vi "Test Basic DAQ.vi"() -> ()   [LabVIEW 2011, in "Diamond Universal Driver.lvlib"]
uses:
  Diamond Universal Driver.lvlib
  Controls/dscBool.ctl
  Controls/board type.ctl
  Controls/dsccb.ctl
  constants.vi
  Controls/gain.ctl
  Controls/dscADSettings.ctl
  Controls/state.ctl
  Controls/dscADScan.ctl
  Controls/dscPolarity.ctl
  Controls/dscDASettings.ctl
panel:
  out "error out 2":errorcluster
  out "error out":errorcluster
  out "LED V":dbl
  out "LED Curr":dbl
  out "P tot":dbl
  out "P up":dbl
  out "T Imp":dbl
  out "RH Imp":dbl
  out "T total":dbl
  out "RH Total":dbl
  out "T Upstream":dbl
  out "RH  Upstream":dbl
  out "purge flow":dbl
  out "sample flow":dbl
  out "sheath flow":dbl
  in  "LED On":bool
  in  "Inlet Temp":dbl
  in  "Purge Flow":dbl
  in  "Samp Flow":dbl
  in  "Sheath Flow":dbl
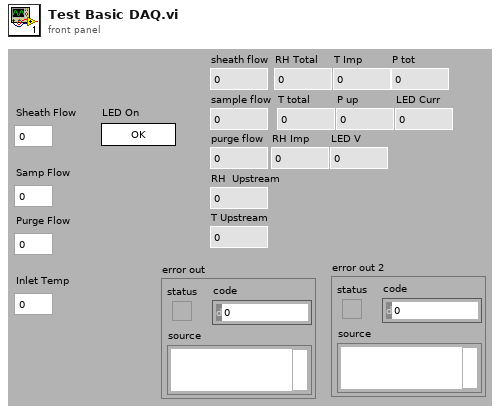
[diagram p1: front panel]
types:
  T1 = typedef "Diamond Universal Driver.lvlib/dscDASettings.ctl" = cluster{"polarity":T2, "load_cal":T3, "range":sgl, "Gain":enum16{"Gain of 1", "Gain of 2", "Gain of 4", "Gain of 8"}, "daSim":u8, "daPolEn":u8, "daUR":u8, "daURCh":u8}
  T2 = typedef "Diamond Universal Driver.lvlib/dscPolarity.ctl" = enum8{"BIPOLAR", "UNIPOLAR"}
  T3 = typedef "dscBool.ctl" = i32
  T4 = typedef "Diamond Universal Driver.lvlib/state.ctl" = enum16{"Sample", "Wait"}
  T5 = typedef "dscADSettings.ctl" = cluster{"current_ch":u8, "gain":T6, "range":enum8{"RANGE_5", "RANGE_10"}, "polarity":enum16{"BIPOLAR", "UNIPOLAR"}, "load cal":u8, "scan_int":enum8{"20", "15", "10", "5", "9", "4"}, "addiff":enum8{"Single Ended", "Differential"}}
  T6 = typedef "gain.ctl" = enum8{"GAIN_1", "GAIN_2", "GAIN_8"}
  T7 = typedef "board type.ctl" = u8
  T8 = typedef "dsccb.ctl" = cluster{"board type":T7, "board num":i16, "base addr":u16, "int level":u8, "RMM external trig":T3, "RMM external trig c3":T3, "EMM IOAdd":u16[], "EMM IOInterrupt":u16[], "clkfreq0":enum8{"10 MHz", "1 MHz"}, "clkfreq1":enum8{"10 MHz", "1 MHz"}, "clksel1":enum8{"Internal (clkfrq1)", "External"}, "address space":dbl, "DAC cfg":u8, "clck_freq":i32, "dma_level":u8, "int_lvl 1":u8, "int_lvl 2":u8, "int_lvl 3":u8, "fpga":u16, "smm_ad_res":u8, "RMM mode 16bit":T3, "RMM DAC 0_3 ext en":T3, "RMM DAC 4_7 ext en":T3}
  T9 = typedef "dscADScan.ctl" = cluster{"low channel":u8, "high channel":u8, "sample_val":u16[], "gain":T6}
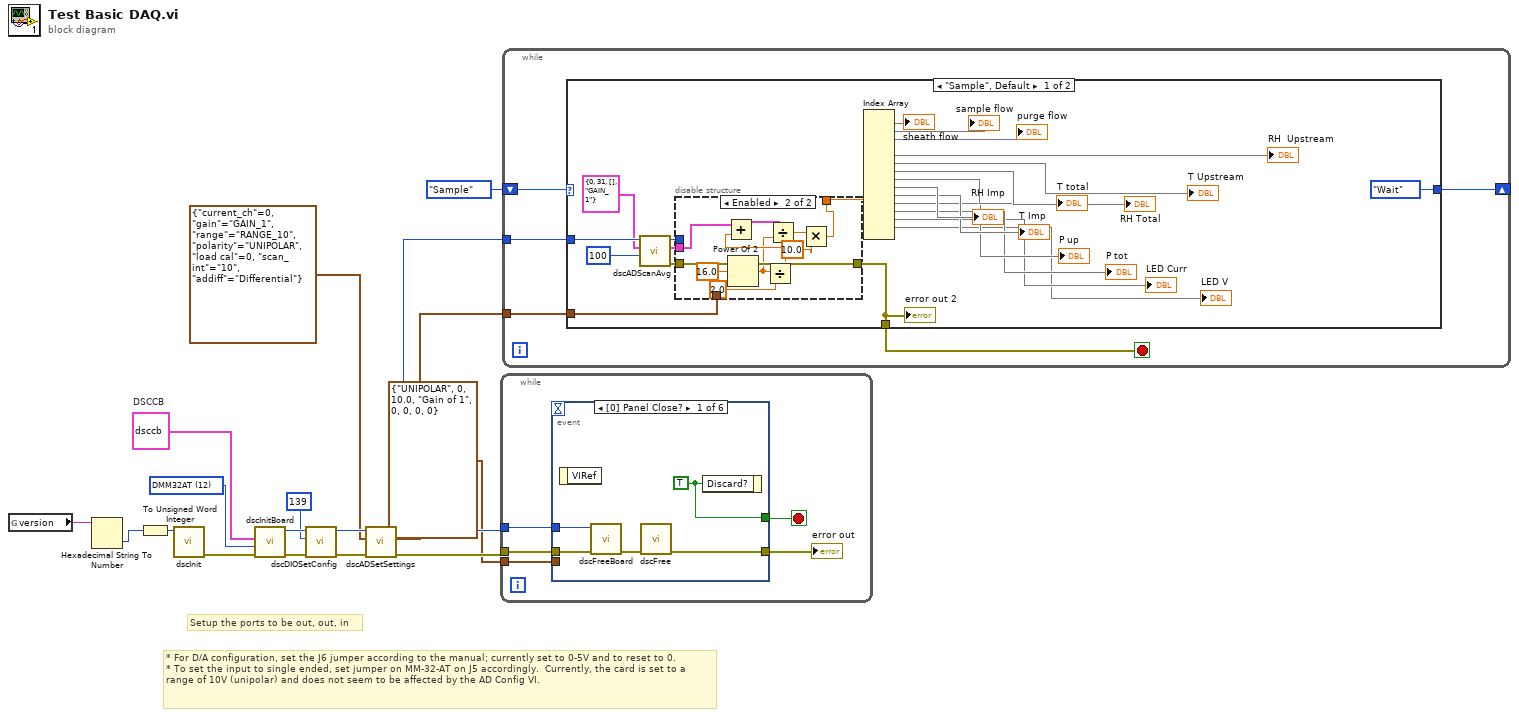
[diagram p0: block diagram]
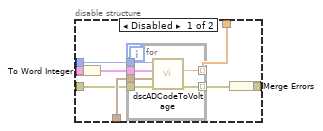
[diagram p2: hidden frame]
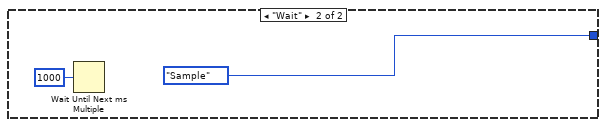
[diagram p3: hidden frame]
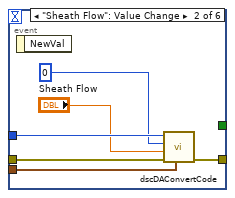
[diagram p4: hidden frame]
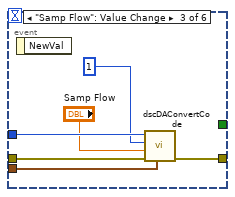
[diagram p5: hidden frame]
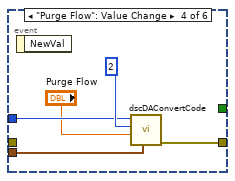
[diagram p6: hidden frame]
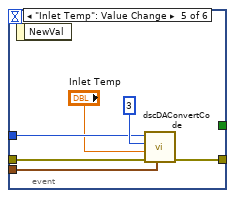
[diagram p7: hidden frame]
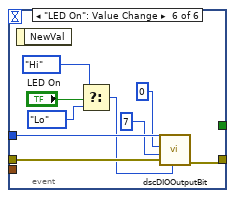
[diagram p8: hidden frame]
diagram:
  w13 = T7 12 items=["DMM16"=0, "RMM"=1, "TMM"=2, "OPMM"=3, "DMM"=4, "SMM"=5, "GMM"=6, "QMM"=7, "ZMM"=8, "PMM"=9, "OMM"=10, "RMM416"=11, "DMM32AT"=12, "EMMDIO"=13, "RMM1612"=14, "DMMAT"=15, "DMM16AT"=16, "IR104"=17, "EMM8"=18, "PROM"=19, "HERCEBX"=20, "CPT"=21, "DMM48AT"=22, "OMMIO"=23, "DIO82C55"=24, "ATHENA"=25, "METIS"=26, "DMM32XAT"=27, "ELEKTRA"=28, "GPIO11_9513"=29, "GPIO11_DIO"=30, "GPIO21"=31, "PSD"=32, "ATHENAII"=33, "DMM32DXAT"=34, "HELIOS"=35, "NEPTUNE"=36, "TEST"=126, "RAW"=127, "DRVR"=255] ("board type")
  w12 = T8 {"board type"=12, "board num"=1, "base addr"=768, "int level"=3, "RMM external trig"=0, "RMM external trig c3"=0, "EMM IOAdd"=[0, 0, 0, 0, 0, 0, 0, 0], "EMM IOInterrupt"=[0, 0, 0, 0, 0, 0, 0, 0], "clkfreq0"=enum."10 MHz", "clkfreq1"=enum."10 MHz", "clksel1"=enum."Internal (clkfrq1)", "address space"=0.0, "DAC cfg"=0, "clck_freq"=0, "dma_level"=0, "int_lvl 1"=0, "int_lvl 2"=0, "int_lvl 3"=0, "fpga"=0, "smm_ad_res"=0, "RMM mode 16bit"=0, "RMM DAC 0_3 ext en"=0, "RMM DAC 4_7 ext en"=0}  # DSCCB
  # "* For D/A configuration, set the J6 jumper according to the manual; currently set to 0-5V and to reset to 0.\n* To set the input to single ended, set jumper on MM-32-AT on J5 accordingly.  Currently, the card is set to a range of 10V (unipolar) and does not seem to be affected by the AD Config VI."
  # "Setup the ports to be out, out, in"
  n1 = global read "constants.vi" "version"() -> (w17:string)
  n2 = Hexadecimal String To Number(string=w17) -> (number=w15:u32)  [unwired: 2 in, 1 out]
  n3 = To Unsigned Word Integer(number=w15) -> (unsigned 16bit integer=w16:u16)
  n4 = call "dscInit.vi"("versionIn"=w16) -> ("error out"=w14:errorcluster)  [unwired: 9 in, 1 out]
  n5 = call "dscInitBoard.vi"("error in"=w14, "board type"=w13, "DSCCB"=w12) -> ("error out"=w10:errorcluster, "boardHandleOut"=w11:i16)  [unwired: 6 in, 1 out]
  n6 = call "dscDIOSetConfig.vi"("error in"=w10, "config_bytes"=u8 139, "board"=w11) -> ("error out"=w7:errorcluster, "boardOut"=w8:i16)  [unwired: 7 in]
  n7 = call "dscADSetSettings.vi"("error in"=w7, "adSettingsIn"=T5 {"current_ch"=0, "gain"=enum."GAIN_1", "range"=enum."RANGE_10", "polarity"=enum."UNIPOLAR", "load cal"=0, "scan_int"=enum."10", "addiff"=enum."Differential"}, "boardIn"=w8) -> ("error out"=w2:errorcluster, "adSettingsOut"=w4:T5, "boardOut"=w3:i16)  [unwired: 6 in]
  n8 = while {
    tunnel: w3 -> [w20]
    tunnel: w2 -> [w21]
    tunnel: T1 {"polarity"=enum."UNIPOLAR", "load_cal"=0, "range"=10.0, "Gain"=enum."Gain of 1", "daSim"=0, "daPolEn"=0, "daUR"=0, "daURCh"=0} ("dscDASettings") -> [w18]
    stop <- w22 stop-if-true
    n9 = event shown="[0] Panel Close?" {
      selector: _ -> [_ _ _ _ _ _]
      dyn-events: _ -> [_ _ _ _ _ _]
      timeout: _ -> [_ _ _ _ _ _]
      tunnel: [w27 _ _ _ _ _] -> w22
      tunnel: w21 -> [w24 w30 w39 _ w47 w58]
      tunnel: w20 -> [w25 w33 w36 w43 w49 w59]
      tunnel: [w23 w29 w37 w40 w45 w57] -> w19
      tunnel: w18 -> [_ w28 w38 w42 w46 _]
      event Panel Close? {
        w27 = TRUE ("Discard?")
        n10 = event-data() -> ()  [unwired: 1 in, 1 out]
        n11 = call "dscFreeBoard.vi"("error in"=w24, "boardIn"=w25) -> ("error out"=w26:errorcluster)  [unwired: 8 in, 1 out]
        n12 = call "dscFree.vi"("error in"=w26) -> ("error out"=w23:errorcluster)  [unwired: 10 in]
        n13 = event-data("Discard?"=w27) -> ()  [unwired: 1 in, 1 out]
      }
      event "Sheath Flow": Value Change {
        n14 = event-data() -> ()  [unwired: 1 in, 1 out]
        n15 = call "dscDAConvertCode.vi"("dscDASettings"=w28, "error in"=w30, "voltage"="Sheath Flow", "channel"=u8 0, "board"=w33) -> ("error out"=w29:errorcluster)  [unwired: 5 in, 1 out]
      }
      event "Samp Flow": Value Change {
        n16 = event-data() -> ()  [unwired: 1 in, 1 out]
        n17 = call "dscDAConvertCode.vi"("dscDASettings"=w38, "error in"=w39, "voltage"="Samp Flow", "channel"=u8 1, "board"=w36) -> ("error out"=w37:errorcluster)  [unwired: 5 in, 1 out]
      }
      event "Purge Flow": Value Change {
        n18 = event-data() -> ()  [unwired: 1 in, 1 out]
        n19 = call "dscDAConvertCode.vi"("dscDASettings"=w42, "voltage"="Purge Flow", "channel"=u8 2, "board"=w43) -> ("error out"=w40:errorcluster)  [unwired: 6 in, 1 out]
      }
      event "Inlet Temp": Value Change {
        n20 = event-data() -> ()  [unwired: 1 in, 1 out]
        n21 = call "dscDAConvertCode.vi"("dscDASettings"=w46, "error in"=w47, "voltage"="Inlet Temp", "channel"=u8 3, "board"=w49) -> ("error out"=w45:errorcluster)  [unwired: 5 in, 1 out]
      }
      event "LED On": Value Change {
        n22 = event-data() -> ()  [unwired: 1 in, 1 out]
        n23 = Select(t=enum8{"Lo", "Hi"}."Hi", s="LED On", f=enum8{"Lo", "Hi"}."Lo" ("bit_val")) -> (s? t:f=w51:enum8{"Lo", "Hi"})
        n24 = call "dscDIOOutputBit.vi"("bit_val"=w51, "error in"=w58, "bit"=u8 7, "port"=u8 0, "board"=w59) -> ("error out"=w57:errorcluster)  [unwired: 5 in, 1 out]
      }
    }
    "error out" <- w19
  }
  n25 = while {
    tunnel: w3 -> [w63]
    shift-right: [w61] -> _
    shift-left: state."Sample" ("state") -> [w64]
    tunnel: w4 -> [w60]
    stop <- w62 stop-if-true
    n26 = case shown="\"Sample\", Default" w64 {
      tunnel: w63 -> [w87 _]
      tunnel: [w65 _] -> w62
      tunnel: [state."Wait" ("state") state."Sample" ("state")] -> w61
      tunnel: w60 -> [w70 _]
      frame "Sample", Default {
        n27 = call "dscADScanAvg.vi"("count"=100, "dscadscan"=T9 {"low channel"=0, "high channel"=31, "sample_val"=[], "gain"=enum."GAIN_1"}, "board"=w87) -> ("error out"=w66:errorcluster, "DataOut"=w68:cluster{"time":timestamp, "sample_val":sgl[]}, "boardOut"=w69:i16)  [unwired: 6 in]
        n28 = disable-structure shown="Enabled" {
          disable-tunnel: w70 -> [w95 _]
          disable-tunnel: w69 -> [w94 _]
          disable-tunnel: w68 -> [w93 w108]
          disable-tunnel: [w91 w102] -> w67
          disable-tunnel: w66 -> [w90 w111]
          disable-tunnel: [w88 w111] -> w65
          frame Disabled {
            n29 = To Word Integer(number=w93) -> (16bit integer=w92:cluster{"time":i16, "sample_val":i16[]})
            n30 = for {
              tunnel: w95 -> [w101]
              tunnel: w94 -> [w100]
              tunnel: w92 -> [w99]
              tunnel: [w98] -> w91 mode=indexing
              tunnel: w90 -> [w97]
              tunnel: [w96] -> w89 mode=indexing
              n31 = call "dscADCodeToVoltage.vi"("error in"=w97, "AD Settings"=w101, "adCode"=w99, "board"=w100) -> ("error out"=w96:errorcluster, "voltage"=w98:dbl)  [unwired: 4 in, 2 out]
            }
            n32 = Merge Errors(w89) -> (w88:errorcluster)
          }
          frame Enabled {
            n33 = Power Of 2(x=16.0) -> (2^x=w105:dbl)
            n34 = Divide(x=w105, y=2.0) -> (x/y=w107:dbl)
            n35 = Add(x=w108, y=w107) -> (x+y=w106:cluster{"time":timestamp, "sample_val":dbl[]})
            n36 = Divide(x=w106, y=w105) -> (x/y=w104:dbl)
            n37 = Multiply(x=w104, y=10.0) -> (x*y=w102:dbl)
          }
        }
        "error out 2" <- w65
        n38 = Index Array(array=w67) -> (element #1=→"sheath flow", element #2=→"sample flow", element #3=→"purge flow", element #4=→"RH  Upstream", element #5=→"T Upstream", element #6=→"RH Total", element #7=→"T total", element #8=→"RH Imp", element #9=→"T Imp", element #10=→"P up", element #11=→"P tot", element #12=→"LED Curr", element #13=→"LED V")  [unwired: 14 in, 1 out]
      }
      frame "Wait" {
        n39 = Wait Until Next ms Multiple(millisecond multiple=u32 1000) -> ()  [unwired: 1 out]
      }
    }
  }
